vi "Read.vi"(8 "error in (no error)":errorcluster, 11 "IP Connection in":refnum<class "IP Connection.lvclass">) -> (0 "error out":errorcluster, 1 "Function ID":u8, 2 "Stack ID":u8, 3 "IP Connection out":refnum<class "IP Connection.lvclass">, 4 "Data":string, 5 "timed out":bool)   [LabVIEW 2011, in "Tinkerforge.lvlib" / "IP Connection.lvclass"]
doc: "This VI reads a complete message."
uses:
  IP Connection.lvclass
  Type Definitions/Connection Status.ctl
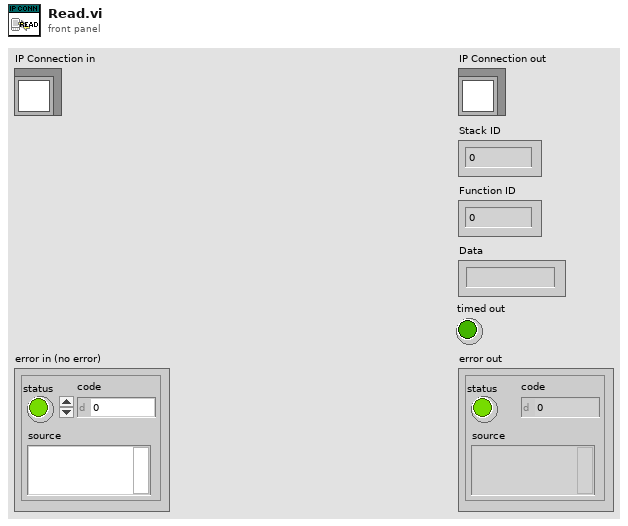
[diagram p1: front panel]
types:
  T1 = enum16{"Standard", "Buffered", "CRLF", "Immediate"}
  T2 = typedef "Tinkerforge.lvlib/IP Connection.lvclass/Connection Status.ctl" = enum16{"Uninitialized", "Connected", "Reconnecting", "Disconnected"}
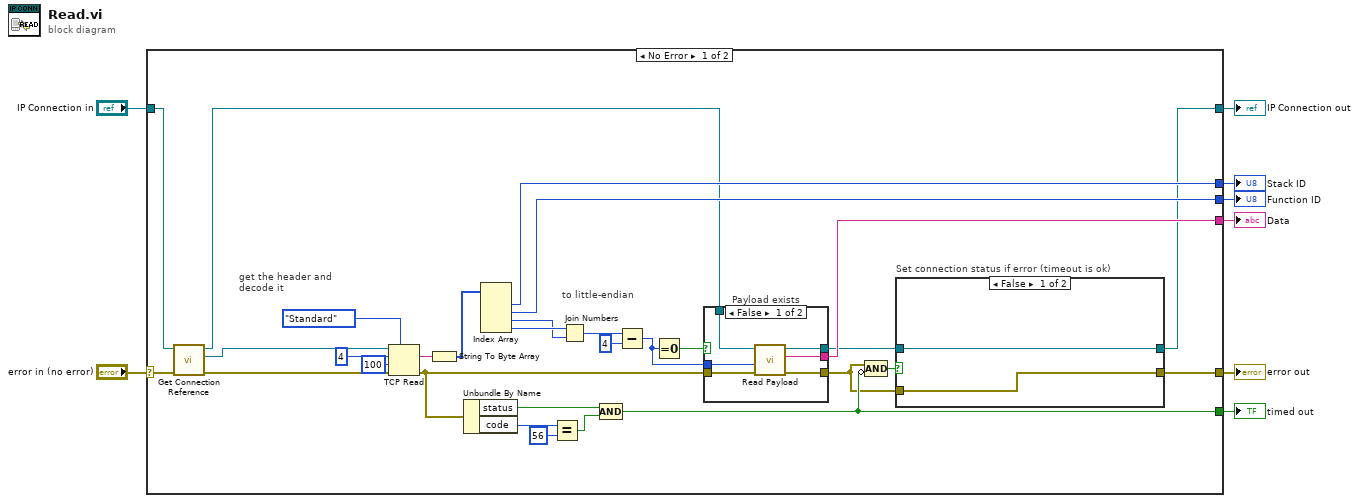
[diagram p0: block diagram]
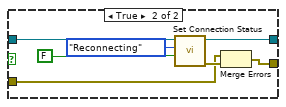
[diagram p2: hidden frame]
diagram:
  n1 = case shown="No Error" "error in (no error)" {
    selector: "error in (no error)" -> [w19 w57]
    tunnel: [w9 w57] -> w7
    tunnel: [w10 w56] -> w5
    tunnel: "IP Connection in" -> [w17 w56]
    tunnel: [w34 _] -> w4
    tunnel: [w33 _] -> w3
    tunnel: [w26 _] -> w2
    tunnel: [w14 _] -> w1
    frame No Error {
      # "to little-endian"
      # "get the header and\ndecode it"
      n2 = call "Get Connection Reference.vi"("error in (no error)"=w19, "IP Connection in"=w17) -> ("error out"=w18:errorcluster, "TCP Network Connection"=w15:refnum<k5>, "IP Connection out"=w16:refnum<class "IP Connection.lvclass">)  [unwired: 7 in]
      n3 = TCP Read(connection ID=w15, bytes to read=4, error in (no error)=w18, 7:T1."Standard" ("mode (standard)"), 9:100 ("timeout ms (25000)")) -> (data out=w36:string, error out=w25:errorcluster)  [unwired: 1 out]
      n4 = String To Byte Array(string=w36) -> (unsigned byte array=w35:u8[])
      n5 = Unbundle By Name(w25) -> ("status"=w21:bool, "code"=w24:i32)
      n6 = Index Array(array=w35) -> (element #1=w34:u8, element #2=w33:u8, element #3=w31:u8, element #4=w32:u8)  [unwired: 4 in]
      n7 = Equal?(x=w24, y=56) -> (x = y?=w22:bool)
      n8 = Join Numbers(hi=w32, lo=w31) -> ((hi.lo)=w30:u16)
      n9 = Compound Arithmetic op=AND(w21, w22) -> (w14:bool)
      n10 = Subtract(x=w30, y=u16 4 ("x")) -> (x-y=w28:u16)
      n11 = Equal To 0?(x=w28) -> (x = 0?=w27:bool)
      n12 = case "Payload exists" shown="False" w27 {
        tunnel: w25 -> [w53 w55]
        tunnel: [w52 w55] -> w12
        tunnel: w28 -> [w51 _]
        tunnel: w16 -> [w50 w54]
        tunnel: [w49 _] -> w26
        tunnel: [w48 w54] -> w11
        frame False {
          n13 = call "Read Payload.vi"("error in (no error)"=w53, "Payload Size"=w51, "IP Connection in"=w50) -> ("error out"=w52:errorcluster, "Data"=w49:string, "IP Connection out"=w48:refnum<class "IP Connection.lvclass">)  [unwired: 6 in]
        }
        frame True {
        }
      }
      n14 = Compound Arithmetic op=AND(w12, invert w14) -> (w13:bool)
      n15 = case "Set connection status if error (timeout is ok)" shown="False" w13 {
        tunnel: [w39 w46] -> w9
        tunnel: w11 -> [w40 w45]
        tunnel: w12 -> [w39 w42]
        tunnel: [w40 w41] -> w10
        frame False {
        }
        frame True {
          n16 = call "Set Connection Status.vi"("connected?"=FALSE, "Connection Status"=Connection_Status."Reconnecting", "IP Connection in"=w45) -> ("error out"=w47:errorcluster, "IP Connection out"=w41:refnum<class "IP Connection.lvclass">)  [unwired: 7 in]
          n17 = Merge Errors(w42, w47) -> (w46:errorcluster)
        }
      }
    }
    frame Error {
    }
  }
  "error out" <- w7
  "IP Connection out" <- w5
  "Stack ID" <- w4
  "Function ID" <- w3
  "Data" <- w2
  "timed out" <- w1
